vi "RestOperatingHours.vi"(8 "Fehler (Eingang, kein Fehler)":errorcluster, 10 "DataFlowIN (Eingang)":T1, 11 "TableName":string) -> (0 "Fehler (Ausgang)":errorcluster, 2 "Calculeted Operating Hours":dbl, 3 "DataFlowIN (Ausgang)":T1)   [LabVIEW 2017]
uses:
  classes/DataCollector.lvclass
  classes/DataHandler.lvclass
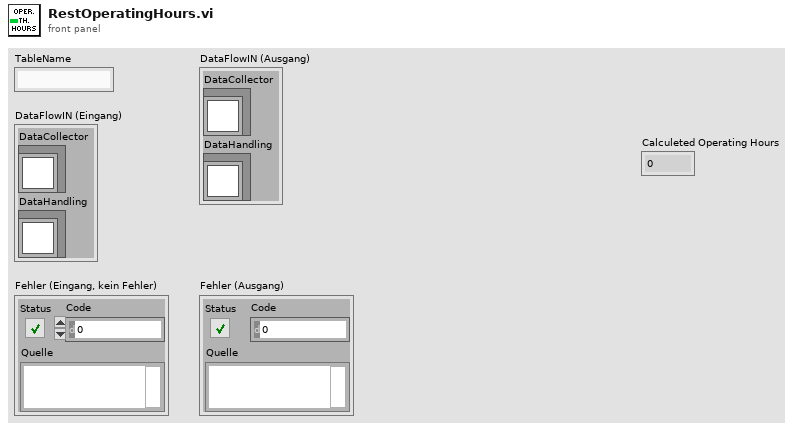
[diagram p1: front panel]
types:
  T1 = cluster{"DataCollector":refnum<class "DataCollector.lvclass">, "DataHandling":refnum<class "DataHandler.lvclass">}
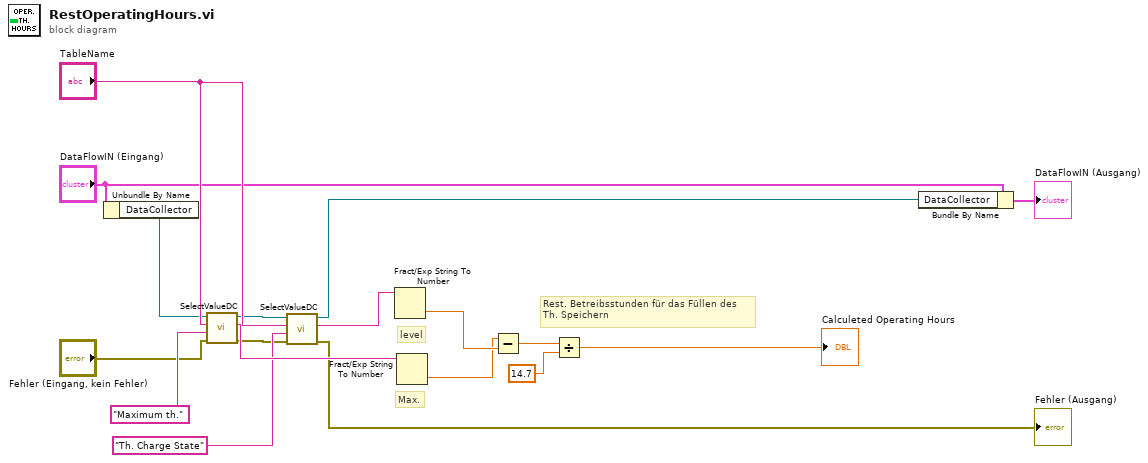
[diagram p0: block diagram]
diagram:
  # "Rest. Betreibsstunden für das Füllen des \nTh. Speichern"
  # "level"
  # "Max."
  n1 = Unbundle By Name("DataFlowIN (Eingang)") -> ("DataCollector"=w8:refnum<class "DataCollector.lvclass">)
  n2 = call-dynamic "SelectValueDC.vi"("error in (no error)"="Fehler (Eingang, kein Fehler)", "Table Row Name"="Maximum th.", "Unique Object Identifier"="TableName", "DataCollector in"=w8) -> ("error out"=w5:errorcluster, "Value"=w14:string, "DataCollector out"=w4:refnum<class "DataCollector.lvclass">)  [unwired: 5 in]
  n3 = call-dynamic "SelectValueDC.vi"("error in (no error)"=w5, "Table Row Name"="Th. Charge State", "Unique Object Identifier"="TableName", "DataCollector in"=w4) -> ("error out"=→"Fehler (Ausgang)":errorcluster, "Value"=w13:string, "DataCollector out"=w12:refnum<class "DataCollector.lvclass">)  [unwired: 5 in]
  n4 = Fract/Exp String To Number(string=w13) -> (number=w16:dbl)  [unwired: 3 in, 1 out]
  n5 = Fract/Exp String To Number(string=w14) -> (number=w15:dbl)  [unwired: 3 in, 1 out]
  n6 = Subtract(x=w15, y=w16) -> (x-y=w17:dbl)
  n7 = Divide(x=w17, y=14.7) -> (x/y=→"Calculeted Operating Hours":dbl)
  n8 = Bundle By Name(cluster="DataFlowIN (Eingang)", "DataCollector"=w12) -> (→"DataFlowIN (Ausgang)":T1)
